vi "Create Folder In Location.vi"(8 "Error In":errorcluster, 10 "Folder Name":string="Missions", 11 "Path To Development Folder":path=path "C:/Robotic Systems/Products/Surveyor/Software/Ground Station/SubVI/Missions/File IO") -> (0 "error out":errorcluster, 3 "Path to Created Folder":path)   [LabVIEW 2014]
doc: "Create a folder in the specified location for development and will create the the same folder the \"Data Folder\" when deployed."
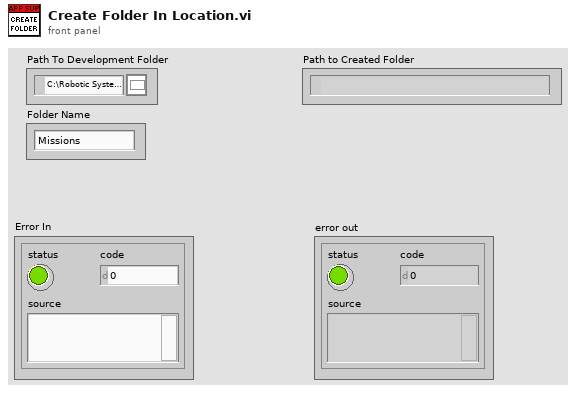
[diagram p1: front panel]
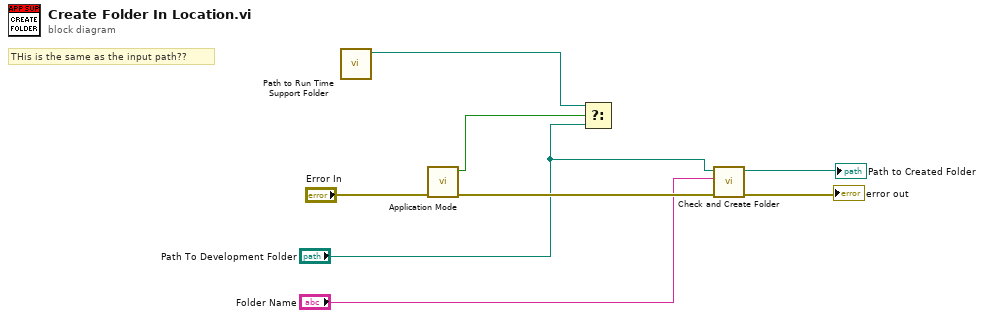
[diagram p0: block diagram]
diagram:
  # "THis is the same as the input path??"
  n1 = call "Path to Run Time Support Folder.vi"() -> ("Path To Run Time Support Folder"=w2:path)  [unwired: 10 in, 1 out]
  n2 = call "Application Mode.vi"("error in (no error)"="Error In") -> ("error out"=w6:errorcluster, "Run Time Mode?"=w8:bool)  [unwired: 9 in]
  n3 = Select(t=w2, s=w8, f="Path To Development Folder") -> ()  [unwired: 1 out]
  n4 = call "Check and Create Folder.vi"("error in"=w6, "Folder Name"="Folder Name", "Path to Directory"="Path To Development Folder") -> ("error out"=→"error out":errorcluster, "Path to Folder"=→"Path to Created Folder":path)  [unwired: 7 in]
